vi "APS read d channel output.vi"(7 "DO_Data":i32, 8 "error in (no error)":errorcluster caption="错误输入（无错误）", 9 "Ch_No":i32, 10 "DO_Group":i32, 11 "Board_ID":i32) -> (0 "error out":errorcluster caption="错误输出", 3 "function return":i32, 5 "DO_Data out":i32)   [LabVIEW 2011, in "APS168.lvlib"]
doc: "I32 FNTYPE APS_read_d_channel_output(I32 Board_ID, I32 DO_Group, I32 Ch_No, I32 *DO_Data);"
uses:
  APS168.lvlib
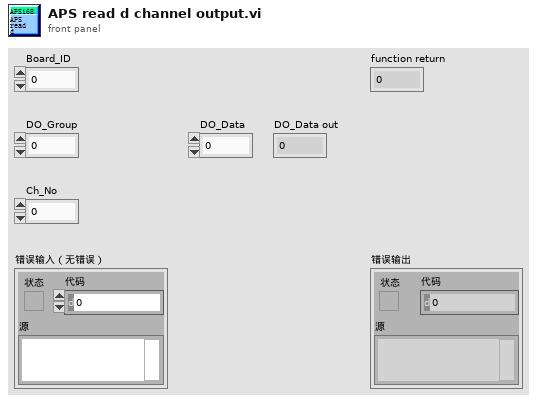
[diagram p1: front panel]
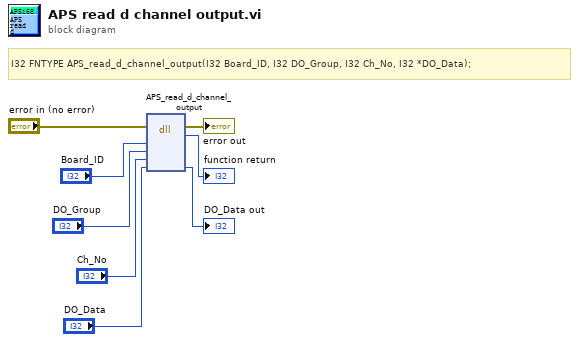
[diagram p0: block diagram]
diagram:
  # "I32 FNTYPE APS_read_d_channel_output(I32 Board_ID, I32 DO_Group, I32 Ch_No, I32 *DO_Data);"
  n1 = dll-call lib="PTH1Labs E软件ADLINK 204CAPS_1_7_1_LIB line 连续运动204APS168.*" fn="APS_read_d_channel_output"(error in="error in (no error)", "Board_ID"="Board_ID", "DO_Group"="DO_Group", "Ch_No"="Ch_No", "DO_Data"="DO_Data") -> (error out=→"error out":errorcluster, →"function return":i32, "DO_Data"=→"DO_Data out":i32)  [unwired: 5 in, 1 out]
